vi "LSMcontroller_v57.vi"() -> ()   [LabVIEW 2015] (continued)
      # "Look in disabled \nchannelselect example next to this\nto understand how channels get propagated \nthrough the progam\n\nthe configuration file contains all\navailable channels in an array.\nat the start of the program lists of available \ninput channels and  menu rings of available output channels are loaded from here.\n\nif you add channels to record from/output to, make sure to expand the channel array in config.\n\nOnce the lists and rings are loaded, items in the list can be selected via click and  shift-click.\nThe ao channels in the ring are added one by one, with a defined waveform.\n\nPropagating through the program in the 2p param buffers are only 4 arrays of numbers, which are the indices of the selected channels from the list in order. \nThus, the index in the active channels array DOES NOT tell you which channel it represents: the actual CONTENT/NUMBER at a particular index in the active channels arrays tells you which channel it represents, since that number is the index in the fixed channel array in config."
      n2 = stacked-sequence {
        frame #0 {
          n3 = call "lifetimeparameters.vi"("command"="clear") -> ()  [unwired: 1 in, 1 out]
          n4 = call "2pparameters.vi"("command"="clear") -> ()  [unwired: 1 in, 1 out]
        }
        frame #1 {
          w39 = TRUE ("auto shutter")
          n5 = call "2pparameters.vi"("command"="get") -> ("params out"=w41:T12)  [unwired: 1 in]
          n6 = Bundle By Name(cluster=w41, "autoshutter"=w39, "auto OD"=w39) -> (w40:T12)
          n7 = local write "auto shutter"(w39) -> ()
          n8 = local write "auto OD"(w39) -> ()
          n9 = call "2pparameters.vi"("Params in"=w40, "command"="set") -> ()  [unwired: 1 out]
        }
        frame #2 {
          # "Disabled Thorlabs Zstage;\nneeds to be replaced by PI code"
          # "Initialize Z-axis controller: Thorlabs MTS25-Z8"
          n10 = disable-structure shown="Disabled" {
            frame Disabled {
              n11 = call "Z-ControllerInterFace.vi"() -> ("motorref"=w45:refnum<k7>)  [unwired: 1 in]
              n12 = call "setmotorparam.vi"("Automation Refnum in"=w45) -> ("motorref out"=w46:refnum<k7>)
              n13 = call "2pparameters.vi"("command"="get") -> ("params out"=w49:T12)  [unwired: 1 in]
              n14 = Bundle By Name(cluster=w49, "motorref"=w46) -> (w50:T12)
              n15 = call "2pparameters.vi"("Params in"=w50, "command"="set") -> ()  [unwired: 1 out]
            }
            frame Enabled {
            }
          }
          n16 = local write "Thorlabs Zstage disabled"(TRUE ("64bit disabled")) -> ()
        }
        frame #3 {
          n17 = call "2pparameters.vi"("command"="get") -> ("params out"=w53:T12)  [unwired: 1 in]
          n18 = Bundle By Name(cluster=w53, "type"="X-Y-t movie") -> (w55:T12)
          n19 = call "2pparameters.vi"("Params in"=w55, "command"="set") -> ()  [unwired: 1 out]
        }
      }
      n20 = property on="Exit" class="Bool (strict)"("Val(Sgnl)"=w24) -> ()  [unwired: 2 in, 2 out]
      n21 = property on="Start" class="Bool (strict)"("Val(Sgnl)"=w24) -> ()  [unwired: 2 in, 2 out]
      n22 = property on="Stop" class="Bool (strict)"("Val(Sgnl)"=w24) -> ()  [unwired: 2 in, 2 out]
      n23 = property on="Start" class="Bool (strict)"("Visible"=TRUE, "DisabledEnum"=T8."Enabled" ("Disabled")) -> ()  [unwired: 2 in, 2 out]
      n24 = property on="ROI" class="Bool (strict)"("DisabledEnum"=T8."Enabled" ("Disabled")) -> ()  [unwired: 2 in, 2 out]
      n25 = property on="ROI" class="Bool (strict)"("Value"=FALSE ("ROI")) -> ()  [unwired: 2 in, 2 out]
      n26 = property on="ROI" class="Bool (strict)"("Visible"=TRUE) -> ()  [unwired: 2 in, 2 out]
      n27 = local read "Measurement"() -> (w12:T5)
      n28 = flat-sequence {
        frame #0 {
          n29 = call "configuration.vi"("command"="set") -> ()  [unwired: 2 in, 2 out]
        }
        frame #1 {
          w57 = u16 1 items=["OD 0"=1, "OD 0.5"=2, "OD 1"=3, "OD 2"=4, "OD 3"=5, "OD 4"=6] ("New ODfilt")
          n30 = call "configuration.vi"("command"="get") -> ("config out"=w60:T13)  [unwired: 2 in, 1 out]
          n31 = local read "ODfilt"() -> (w58:u16)
          n32 = Unbundle By Name(w60) -> ("master data dir"=→"data dir":path)
          n33 = call "filterwheelcontrol_nothorlabslib.vi"("Current OD filt"=w57, "New ODfilt"=w58) -> ()  [unwired: 1 in]
        }
        frame #2 {
          n34 = call "configuration.vi"("command"="get") -> ("config out"=w64:T13)  [unwired: 2 in, 1 out]
          n35 = Unbundle By Name(w64) -> ("AI names"=w63:string[], "CI names"=w62:string[])
          n36 = property on="AI channels" class="LstBox (strict)"("Item Names"=w63) -> ()  [unwired: 2 in, 2 out]
          n37 = property on="CI channels" class="LstBox (strict)"("Item Names"=w62) -> ()  [unwired: 2 in, 2 out]
        }
        frame #3 {
          n38 = call "configuration.vi"("command"="get") -> ("config out"=w73:T13)  [unwired: 2 in, 1 out]
          n39 = Unbundle By Name(w73) -> ("AO names"=w69:string[], "DO names"=w68:string[])
          n40 = call "fill channelselector from array.vi"("channel  names"=w69) -> ("channel selector string and values"=w71:cluster{"String":string, "Value":u16}[])
          n41 = Build Array (concatenate)(w69, w68) -> (w67:string[])
          n42 = call "fill channelselector from array.vi"("channel  names"=w68) -> ("channel selector string and values"=w70:cluster{"String":string, "Value":u16}[])
          n43 = property on="AO channels" class="Ring (strict)"("StringsAndValues[]"=w71) -> ()  [unwired: 2 in, 2 out]
          n44 = call "fill channelselector from array.vi"("channel  names"=w67) -> ("channel selector string and values"=w66:cluster{"String":string, "Value":u16}[])
          n45 = property on="DO channels" class="Ring (strict)"("StringsAndValues[]"=w70) -> ()  [unwired: 2 in, 2 out]
          n46 = property on="refwf" class="Ring (strict)"("StringsAndValues[]"=w66) -> ()  [unwired: 2 in, 2 out]
        }
      }
      n47 = case shown="\"Lifetime (point)\", \"Lifetime (scan)\"" w12 {
        frame "Lifetime (point)", "Lifetime (scan)" {
          n48 = property on="Init" class="Bool (strict)"("Visible"=TRUE, "DisabledEnum"=T8."Enabled" ("Disabled")) -> ()  [unwired: 2 in, 2 out]
          n49 = property on="Start" class="Bool (strict)"("Visible"=FALSE, "DisabledEnum"=T8."Disabled and Grayed Out" ("Disabled")) -> ()  [unwired: 2 in, 2 out]
        }
        frame "X-Y-t movie", Default {
        }
      }
      n50 = call "seterrors.vi"("error IO"=errorcluster {"status"=FALSE, "code"=0, "source"=""}) -> ()
      n51 = property on="Stop" class="Bool (strict)"("Visible"=FALSE, "DisabledEnum"=T8."Disabled and Grayed Out" ("Disabled")) -> ()  [unwired: 2 in, 2 out]
      n52 = property on="Init" class="Bool (strict)"("Visible"=FALSE, "DisabledEnum"=T8."Disabled and Grayed Out" ("Disabled")) -> ()  [unwired: 2 in, 2 out]
      n53 = Current VI's Path() -> (path=w10:path)
      n54 = Strip Path(path=w10) -> (stripped path=w11:path)  [unwired: 1 out]
      n55 = Build Path(base path=w11, name or relative path="LaserControl.vi") -> (appended path=w9:path)
      n56 = call "loadcolormaps.vi"() -> ()  [unwired: 12 in]
      n57 = stacked-sequence {
        frame #0 {
          n58 = call "waveformsDObuffer.vi"("command"="clear") -> ()  [unwired: 1 in, 1 out]
          n59 = call "waveformsAObuffer.vi"("command"="clear") -> ()  [unwired: 1 in, 1 out]
        }
        frame #1 {
          n60 = call "Used AO lines.vi"() -> ("used AO names"=w27:string[], "used AO lines"=w29:tag[])  [unwired: 2 in]
          n61 = control-ref of="Analog Lines Plot"() -> (w28:refnum<vi>)
          n62 = local write "Analog Used Lines"(w29) -> ()
          n63 = local write "Analog Used Names"(w27) -> ()
          n64 = call "prepAOWaveplot.vi"("WaveformGraph in"=w28, "Analog Used Names"=w27) -> ()  [unwired: 1 in]
          n65 = control-ref of="Digital Lines Plot"() -> (w30:refnum<vi>)
          n66 = call "Used DO lines.vi"() -> ("used DO names"=w31:string[], "used DO lines"=w32:tag[])  [unwired: 2 in]
          n67 = local write "Digital Used Lines"(w32) -> ()
          n68 = local write "Digital Used Names"(w31) -> ()
          n69 = call "prepDOWaveplot.vi"("DigitalGraph in"=w30, "used DO names"=w31) -> ()  [unwired: 1 in]
        }
      }
      n70 = Open VI Reference(type specifier VI Refnum (for type only)=refnum<vi> refnum, vi path=w9, options=128) -> (vi reference=w2:refnum<vi>, error out=w6:errorcluster)  [unwired: 3 in]
      n71 = call-by-ref "Start Asynchronous Call"(reference=w2, error in=w6) -> (reference out=w7:refnum<vi>, error out=w5:errorcluster)  [unwired: 12 in]
      n72 = Close Reference(reference=w7, error in (no error)=w5) -> ()  [unwired: 1 out]
      n73 = disable-structure shown="Enabled" {
        frame Disabled {
          n74 = call "channelselectexample.vi"() -> ()  [unwired: 12 in]
        }
        frame Enabled {
        }
      }
      "ROI Type" <- w15
    }
    frame #2 {
      n75 = while {
        stop <- w2050 stop-if-true
        n76 = event shown="[15] \"readpatch\": Value Change" {
          selector: _ -> [_ _ _ _ _ _ _ _ _ _ _ _ _ _ _ _ _ _ _ _ _ _ _ _ _ _ _ _ _ _ _ _ _ _ _ _ _ _ _ _ _]
          dyn-events: _ -> [_ _ _ _ _ _ _ _ _ _ _ _ _ _ _ _ _ _ _ _ _ _ _ _ _ _ _ _ _ _ _ _ _ _ _ _ _ _ _ _ _]
          timeout: _ -> [_ _ _ _ _ _ _ _ _ _ _ _ _ _ _ _ _ _ _ _ _ _ _ _ _ _ _ _ _ _ _ _ _ _ _ _ _ _ _ _ _]
          tunnel: [_ _ _ _ _ _ _ _ _ _ _ _ _ _ _ _ _ _ _ _ _ _ _ _ _ _ _ _ _ _ _ _ _ _ _ _ _ _ _ _ "Exit"] -> w2050
          event "Start": Value Change {
            n77 = event-data() -> ()  [unwired: 1 in, 5 out]
            n78 = local read "Start"() -> (w2051:bool)
            n79 = case shown="True" w2051 {
              frame False {
              }
              frame True {
                # "X"
                # "Y"
                n80 = local read "Measurement"() -> (w2052:T5)
                n81 = case shown="\"Timetrace\", \"Lifetime (contour)\"" w2052 {
                  frame "X-Y-t movie", "X-Y-Z stack", "Lifetime (scan)" {
                    n82 = stacked-sequence {
                      seq-local: [_ w2094 _ _ _ _ _ _ _ _ _ _ _] -> [_ _ _ w2947 _ _ _ w2979 w3156 _ _ w3566 _]
                      seq-local: [_ w2092 _ _ _ _ _ _ _ _ _ _ _] -> [_ _ _ _ _ _ _ _ _ _ w3256 _ _]
                      seq-local: [_ w2091 _ _ _ _ _ _ _ _ _ _ _] -> [_ _ _ _ _ _ _ _ _ _ w3255 _ _]
                      seq-local: [_ w2090 _ _ _ _ _ _ _ _ _ _ _] -> [_ _ _ _ _ _ _ _ _ _ w3254 _ _]
                      seq-local: [_ w2089 _ _ _ _ _ _ _ _ _ _ _] -> [_ _ _ _ _ _ _ _ _ _ w3253 _ _]
                      seq-local: [_ w2088 _ _ _ _ _ _ _ _ _ _ _] -> [_ _ _ _ _ _ _ _ _ _ w3252 _ _]
                      seq-local: [_ w2087 _ _ _ _ _ _ _ _ _ _ _] -> [_ _ _ _ _ _ _ _ _ _ w3251 _ _]
                      seq-local: [_ w2086 _ _ _ _ _ _ _ _ _ _ _] -> [_ _ _ _ _ _ _ _ _ _ w3246 _ _]
                      seq-local: [_ w2085 _ _ _ _ _ _ _ _ _ _ _] -> [_ _ _ _ _ _ _ _ _ _ w3245 _ _]
                      seq-local: [_ w2084 _ _ _ _ _ _ _ _ _ _ _] -> [_ _ _ _ _ _ _ _ _ _ w3250 _ _]
                      seq-local: [_ w2083 _ _ _ _ _ _ _ _ _ _ _] -> [_ _ _ _ _ _ _ _ _ _ w3249 _ _]
                      seq-local: [_ w2081 _ _ _ _ _ _ _ _ _ _ _] -> [_ _ _ _ _ _ _ _ _ _ w3244 _ _]
                      seq-local: [_ w2082 _ _ _ _ _ _ _ _ _ _ _] -> [_ _ _ _ _ _ _ _ _ _ w3243 _ _]
                      seq-local: [_ w2080 _ _ _ _ _ _ _ _ _ _ _] -> [_ _ _ _ _ _ _ _ _ _ w3247 _ _]
                      seq-local: [_ w2079 _ _ _ _ _ _ _ _ _ _ _] -> [_ _ _ _ _ _ _ _ _ _ w3248 _ _]
                      frame #0 {
                        w2053 = u16 0 items=["Image", "Rectangle", "Circle", "Freeform Boundary", "Freeform Interior", "Ellipse Boundary", "Line"] ("ROI Type")
                        n83 = local read "finite samples"() -> (w2054:bool)
                        n84 = case shown="True" w2054 {
                          frame False {
                          }
                          frame True {
                            n85 = local read "# of frames"() -> (w2055:i32)
                            n86 = Greater?(x=w2055, y=999) -> (0:w2056:bool)
                            n87 = case shown="True" w2056 {
                              tunnel: w2055 -> [_ w2060]
                              frame False {
                              }
                              frame True {
                                n88 = flat-sequence {
                                tunnel: w2060 -> [w2061]
                                tunnel: [w2062] -> w2059
                                tunnel: [w2061] -> w2058
                                tunnel: w2059 -> [w2074]
                                tunnel: w2058 -> [w2073]
                                frame #0 {
                                n89 = Number To Decimal String(number=w2061) -> (decimal integer string=w2066:string)  [unwired: 1 in]
                                n90 = Concatenate Strings("Yes: record " ("Left Button Text (\"Yes\")"), w2066, " frames" ("string")) -> (w2067:string)
                                n91 = Concatenate Strings("# of frames is " ("message"), w2066, ". Did you mean to do that?" ("string")) -> (w2069:string)
                                n92 = call <vilib>:"Three Button Dialog.vi"("Allow user to close window? (TRUE)"=FALSE, "Right Button Text (\"Cancel\")"="no: record 10 frames" ("Right Button Text (\"Cancel\")"), "Center Button Text (\"No\")"="No: record 1 frame" ("Center Button Text (\"No\")"), "Left Button Text (\"Yes\")"=w2067, "message"=w2069) -> ("Which Button?"=w2062:T14)  [unwired: 6 in]
                                }
                                frame #1 {
                                n93 = case shown="\"Window Close\"" w2074 {
                                tunnel: w2073 -> [w2075 _ _ _]
                                frame "Left Button" {
                                n94 = local write "# of frames"(w2075) -> ()
                                }
                                frame "Center Button", Default {
                                n95 = local write "# of frames"(1 ("# of frames")) -> ()
                                }
                                frame "Right Button" {
                                n96 = local write "# of frames"(10 ("# of frames")) -> ()
                                }
                                frame "Window Close" {
                                n97 = local write "# of frames"(1 ("# of frames")) -> ()
                                }
                                }
                                }
                                }
                              }
                            }
                          }
                        }
                        n98 = local write "ROI Type"(w2053) -> ()
                      }
                      frame #1 {
                        # "change active waveform numbers array"
                        n99 = local read "save\ndata"() -> (w2093:bool)
                        n100 = Get Date/Time In Seconds() -> (seconds since 1Jan1904=w2095:timestamp)
                        n101 = case shown="True" w2093 {
                          tunnel: w2095 -> [w2096 w2098]
                          tunnel: [w2096 w2097] -> w2094
                          frame False {
                          }
                          frame True {
                            n102 = call "createdatafolder.vi"("timestamp in"=w2098) -> ("current data path"=w2099:path, "timestamp out"=w2097:timestamp)
                            n103 = local write "data dir"(w2099) -> ()
                          }
                        }
                        n104 = stacked-sequence {
                          tunnel: w2094 -> [_ w2106 _ _ _ _ _ _ _ _]
                          tunnel: [_ _ _ _ _ w2249 _ _ _ _] -> w2092
                          tunnel: [_ _ _ _ _ w2248 _ _ _ _] -> w2091
                          tunnel: [_ _ _ _ _ w2247 _ _ _ _] -> w2090
                          tunnel: [_ _ _ _ _ w2246 _ _ _ _] -> w2089
                          tunnel: [_ _ _ _ _ w2245 _ _ _ _] -> w2088
                          tunnel: [_ _ _ _ _ w2244 _ _ _ _] -> w2087
                          tunnel: [_ _ _ _ _ w2243 _ _ _ _] -> w2086
                          tunnel: [_ _ _ _ _ w2242 _ _ _ _] -> w2085
                          tunnel: [_ _ _ _ _ w2241 _ _ _ _] -> w2084
                          tunnel: [_ _ _ _ _ w2240 _ _ _ _] -> w2083
                          tunnel: [_ _ _ _ _ w2239 _ _ _ _] -> w2082
                          tunnel: [_ _ _ _ _ w2238 _ _ _ _] -> w2081
                          tunnel: [_ _ _ _ _ w2237 _ _ _ _] -> w2080
                          tunnel: [_ _ _ _ _ w2236 _ _ _ _] -> w2079
                          frame #0 {
                            n105 = local read "AI channels"() -> (w2105:i32[])
                            n106 = local read "CI channels"() -> (w2104:i32[])
                            n107 = call "2pparameters.vi"("command"="get") -> ("params out"=w2102:T12)  [unwired: 1 in]
                            n108 = Bundle By Name(cluster=w2102, "aAI"=w2105, "aCI"=w2104) -> (w2103:T12)
                            n109 = call "2pparameters.vi"("Params in"=w2103, "command"="set") -> ()  [unwired: 1 out]
                          }
                          frame #1 {
                            n110 = local read "Vy-min ref"() -> (w2110:dbl)
                            n111 = local read "Vy-max ref"() -> (w2111:dbl)
                            n112 = local read "Angle ref"() -> (w2109:dbl)
                            n113 = local read "Vx-min ref"() -> (w2112:dbl)
                            n114 = local write "counts"(0 ("counts")) -> ()
                            n115 = local write "graphtab"(T6."image" ("graphtab")) -> ()
                            n116 = local read "Vx-max ref"() -> (w2113:dbl)
                            n117 = property on="Stop" class="Bool (strict)"("Visible"=TRUE, "DisabledEnum"=T8."Enabled" ("Disabled")) -> ()  [unwired: 2 in, 2 out]
                            n118 = property on="Start" class="Bool (strict)"("Visible"=FALSE, "DisabledEnum"=T8."Disabled and Grayed Out" ("Disabled")) -> ()  [unwired: 2 in, 2 out]
                            n119 = script code="Xic=(ximax+ximin)./2;\nYic=(yimax+yimin)./2;\nximin=ximin-Xic;\nymin=ymin-Yic;\nxirmin=ximin.*cos(pi/180.*phi)+yimin.*sin(pi./180.*phi)+Xic;\nyirmin=-ximin.*sin(pi./180.*phi)+yimin.*cos(pi./180.*phi)+Yic;"("ximax"=w2113, "ximin"=w2112, "yimax"=w2111, "yimin"=w2110, "phi"=w2109) -> ("xirmin"=w2108:dbl, "yirmin"=w2107:dbl)  [unwired: 1 in, 1 out]
                            n120 = stacked-sequence {
                              tunnel: w2106 -> [_ w2138 _]
                              frame #0 {
                                n121 = local read "Measurement"() -> (w2120:T5)
                                n122 = case shown="\"X-Y-Z stack\"" w2120 {
                                frame "X-Y-t movie", Default {
                                n123 = call "2pparameters.vi"("command"="get") -> ("params out"=w2123:T12)  [unwired: 1 in]
                                n124 = Bundle By Name(cluster=w2123, "type"="X-Y-t movie") -> (w2121:T12)
                                n125 = call "2pparameters.vi"("Params in"=w2121, "command"="set") -> ()  [unwired: 1 out]
                                }
                                frame "X-Y-Z stack" {
                                n126 = call "2pparameters.vi"("command"="get") -> ("params out"=w2128:T12)  [unwired: 1 in]
                                n127 = Bundle By Name(cluster=w2128, "type"="X-Y-Z stack") -> (w2126:T12)
                                n128 = call "2pparameters.vi"("Params in"=w2126, "command"="set") -> ()  [unwired: 1 out]
                                }
                                frame "Lifetime (scan)" {
                                n129 = call "2pparameters.vi"("command"="get") -> ("params out"=w2133:T12)  [unwired: 1 in]
                                n130 = Bundle By Name(cluster=w2133, "type"="Lifetime (scan)") -> (w2131:T12)
                                n131 = call "2pparameters.vi"("Params in"=w2131, "command"="set") -> ()  [unwired: 1 out]
                                }
                                }
                              }
                              frame #1 {
                                n132 = Format Date/Time String(time format string (%c)="%Y%m%d", seconds (now)=w2138) -> (date/time string=w2137:string)  [unwired: 1 in]
                                n133 = Format Date/Time String(time format string (%c)="%H%M%S", seconds (now)=w2138) -> (date/time string=w2136:string)  [unwired: 1 in]
                                n134 = call "2pparameters.vi"("command"="get") -> ("params out"=w2142:T12)  [unwired: 1 in]
                                n135 = Bundle By Name(cluster=w2142, "date"=w2137, "time"=w2136) -> (w2141:T12)
                                n136 = call "2pparameters.vi"("Params in"=w2141, "command"="set") -> ()  [unwired: 1 out]
                              }
                              frame #2 {
                                n137 = call "configuration.vi"("command"="get") -> ("config out"=w2152:T13)  [unwired: 2 in, 1 out]
                                n138 = Unbundle By Name(w2152) -> ("CI names"=w2153:string[], "AI names"=w2154:string[])
                                n139 = call "2pparameters.vi"("command"="get") -> ("params out"=w2148:T12)  [unwired: 1 in]
                                n140 = Unbundle By Name(w2148) -> ("aCI"=w2149:i32[], "aAI"=w2150:i32[])
                                n141 = for {
                                tunnel: w2149 -> [w2164] mode=indexing
                                tunnel: w2153 -> [w2165]
                                tunnel: [w2163] -> w2155 mode=indexing
                                n142 = Index Array(array=w2165, index=w2164) -> (element=w2163:string)
                                }
                                n143 = for {
                                tunnel: w2150 -> [w2161] mode=indexing
                                tunnel: w2154 -> [w2162]
                                tunnel: [w2160] -> w2156 mode=indexing
                                n144 = Index Array(array=w2162, index=w2161) -> (element=w2160:string)
                                }
                                n145 = Build Array (concatenate)(w2155, w2156) -> (w2146:string[])
                                n146 = for {
                                tunnel: w2146 -> [w2158] mode=indexing
                                tunnel: [w2157] -> w2145 mode=indexing
                                i -> [w2159]
                                n147 = Bundle("String"=w2158, w2159) -> (w2157:cluster{"String":string, i32})  [unwired: 1 in]
                                }
                                n148 = property on="image1list" class="Ring (strict)"("StringsAndValues[]"=w2145) -> ()  [unwired: 2 in, 2 out]
                                n149 = property on="image2list" class="Ring (strict)"("StringsAndValues[]"=w2145) -> ()  [unwired: 2 in, 2 out]
                              }
                            }
                            n150 = call "setposition.vi"("Vy"=w2107, "Vx"=w2108) -> ()  [unwired: 1 in]
                          }
                          frame #2 {
                            n151 = call "X-array-databuffer.vi"("command"=enum16{"get", "set", "clear", "append"}."clear") -> ()  [unwired: 3 in, 2 out]
                            n152 = call "Y-array-databuffer.vi"("command"=enum16{"get", "set", "clear", "append"}."clear") -> ()  [unwired: 3 in, 2 out]
                            n153 = call "2pparameters.vi"("command"="get") -> ("params out"=w2168:T12)  [unwired: 1 in]
                            n154 = Unbundle By Name(w2168) -> ("autoshutter"=w2169:bool, "auto OD"=w2166:bool)
                            n155 = call "allAI-temp_img.vi"("command"=enum16{"get", "set", "clear", "append"}."clear") -> ()  [unwired: 3 in, 2 out]
                            n156 = case shown="True" w2166 {
                              frame False {
                              }
                              frame True {
                                n157 = call "configuration.vi"("command"="get") -> ("config out"=w2177:T13)  [unwired: 2 in, 1 out]
                                n158 = Unbundle By Name(w2177) -> ("image OD"=w2178:u16)
                                n159 = local read "ODfilt"() -> (w2175:u16)
                                n160 = call "filterwheelcontrol_nothorlabslib.vi"("Current OD filt"=w2175, "New ODfilt"=w2178) -> ()  [unwired: 1 in]
                              }
                            }
                            n161 = case shown="True" w2169 {
                              frame False {
                              }
                              frame True {
                                n162 = call "shuttercontrol.vi"("command"="close") -> ()  [unwired: 1 in, 1 out]
                              }
                            }
                            n163 = call "CH1-temp.vi"("command"=enum16{"get", "set", "clear", "add row"}."clear") -> ()  [unwired: 3 in, 2 out]
                            n164 = call "CH2-temp.vi"("command"=enum16{"get", "set", "clear", "add row"}."clear") -> ()  [unwired: 3 in, 2 out]
                          }
                          frame #3 {
                            n165 = local read "avpp"() -> (w2212:i32)
                            n166 = local read "Angle ref"() -> (w2211:dbl)
                            n167 = local read "ROI Type"() -> (w2210:u16)
                            n168 = local read "xpixels ref"() -> (w2207:i32)
                            n169 = local read "Vx-min ref"() -> (w2206:dbl)
                            n170 = local read "Vx-max ref"() -> (w2205:dbl)
                            n171 = local read "ypixels ref"() -> (w2203:i32)
                            n172 = local read "Vy-min ref"() -> (w2204:dbl)
                            n173 = local read "Vy-max ref"() -> (w2200:dbl)
                            n174 = local read "Sampling rate"() -> (w2194:dbl)
                            n175 = local read "finite samples"() -> (w2195:bool)
                            n176 = local read "continuous"() -> (w2198:bool)
                            n177 = local read "wavdet"() -> (w2199:bool)
                            n178 = local read "# of frames"() -> (w2197:i32)
                            n179 = local read "maxbufferAI"() -> (w2196:i32)
                            n180 = local read "Override AI buffer"() -> (w2180:bool)
                            n181 = call "2pparameters.vi"("command"="get") -> ("params out"=w2209:T12)  [unwired: 1 in]
                            n182 = Bundle By Name(cluster=w2209, "avpp"=w2212, "Angle Img"=w2211, "Xpixels Img"=w2207, "Vx-min Img"=w2206, "VX-max Img"=w2205, "Ypixels Img"=w2203, "Vy-min Img"=w2204, "Vy-max Img"=w2200, "srate"=w2194, "srate Img"=w2194, "finite"=w2195, "cont"=w2198, "wavdet"=w2199, "measpoints"=w2197, "maxbufferAI"=w2196, "Drawing Mode"=w2210, "Vz-reset"=0.0, "AIoverride"=w2180) -> (w2201:T12)
                            n183 = call "2pparameters.vi"("Params in"=w2201, "command"="set") -> ()  [unwired: 1 out]
                            n184 = local read "Vholding (mV)"() -> (w2183:sgl)
                            n185 = local read "Current Clamp"() -> (w2189:bool)
                            n186 = local read "Voltage Clamp"() -> (w2188:bool)
                            n187 = local read "OCgain"() -> (w2184:sgl)
                            n188 = local read "CC_ICgain"() -> (w2187:dbl)
                            n189 = local read "holdon"() -> (w2182:bool)
                            n190 = call "patchparameters.vi"("command"="get") -> ("Params out"=w2191:T15)  [unwired: 1 in]
                            n191 = Bundle By Name(cluster=w2191, "VC"=w2188, "CC"=w2189, "CC_icg (pA/mv)"=w2187, "VC_icg (mV/mV)"=sgl 10.0, "OCG (mV/pA)"=w2184, "OVG (mV/mV)"=0.1, "Vhold (mV)"=w2183, "holdon"=w2182) -> (w2190:T15)
                            n192 = call "patchparameters.vi"("Params in"=w2190, "command"="set") -> ()  [unwired: 1 out]
                          }
                          frame #4 {
                            # "Generate Waveforms for Scanning Mirrors"
                            n193 = call "2pparameters.vi"("command"="get") -> ("params out"=w2227:T12)  [unwired: 1 in]
                            n194 = Unbundle By Name(w2227) -> ("srate Img"=w2226:sgl, "Angle Img"=w2225:dbl, "VX-max Img"=w2224:dbl, "Vx-min Img"=w2223:dbl, "Xpixels Img"=w2222:i32, "Ypixels Img"=w2221:i32, "Vy-max Img"=w2220:dbl, "Vy-min Img"=w2219:dbl, "Drawing Mode"=w2218:u16)
                            n195 = call "ROI-databuffer.vi"("command"=enum16{"get", "set", "clear", "append"}."get") -> ("array out"=w2217:cluster{"x":sgl, "y":sgl}[])  [unwired: 4 in]
                            n196 = call "ScanningWaveform_v4.vi"("Vy-min"=w2219, "Vy-max"=w2220, "yPixels/tPixels"=w2221, "xPixels/rPixels"=w2222, "Vx-min"=w2223, "Vx-max"=w2224, "Drawing Mode"=w2218, "Angle"=w2225, "AOrate"=w2226, "Points"=w2217) -> ("numPixels"=w2213:dbl, "Y-WaveArray"=w2216:dbl[], "P"=w2214:dbl, "X-WaveArray"=w2215:dbl[])  [unwired: 6 in]
                            n197 = call "2pparameters.vi"("command"="get") -> ("params out"=w2235:T12)  [unwired: 1 in]
                            n198 = call "Y-array-databuffer.vi"("array in"=w2216, "command"=enum16{"get", "set", "clear", "append"}."set") -> ()  [unwired: 2 in, 2 out]
                            n199 = call "X-array-databuffer.vi"("array in"=w2215, "command"=enum16{"get", "set", "clear", "append"}."set") -> ()  [unwired: 2 in, 2 out]
                            n200 = Bundle By Name(cluster=w2235, "P"=w2214, "sAOxy"=w2213) -> (w2232:T12)
                            n201 = call "2pparameters.vi"("Params in"=w2232, "command"="set") -> ()  [unwired: 1 out]
                          }
                          frame #5 {
                            # "rem2Ps"
                            # "A2Ps"
                            # "Al"
                            # "Rl"
                            n202 = stacked-sequence {
                              seq-local: [w2254 _ _ _ _ _ _ _ _ _ _] -> [_ w2366 _ w2421 _ w2501 _ _ _ _ _]
                              seq-local: [w2255 _ _ _ _ _ _ _ _ _ _] -> [_ w2367 w2377 _ w2470 _ _ _ _ _ _]
                              seq-local: [_ _ w2376 _ _ _ _ _ _ _ _] -> [_ _ _ _ w2464 _ _ _ _ _ _]
                              seq-local: [_ _ _ w2420 _ _ _ _ _ _ _] -> [_ _ _ _ _ w2500 _ _ _ _ _]
                              seq-local: [w2251 _ _ _ _ _ _ _ _ _ _] -> [_ w2363 _ _ _ _ _ _ w2686 w2754 _]
                              seq-local: [w2250 _ _ _ _ _ _ _ _ _ _] -> [_ w2362 _ _ _ _ _ _ w2687 w2755 _]
                              seq-local: [w2257 _ _ _ _ _ _ _ _ _ _] -> [_ _ _ _ _ _ w2539 _ w2685 w2753 _]
                              seq-local: [w2253 _ _ _ _ _ _ _ _ _ _] -> [_ w2361 _ _ _ _ w2538 w2606 _ _ _]
                              seq-local: [w2252 _ _ _ _ _ _ _ _ _ _] -> [_ w2360 _ _ _ _ w2537 w2605 _ _ _]
                              seq-local: [w2256 _ _ _ _ _ _ _ _ _ _] -> [_ _ _ _ _ _ w2536 w2604 _ _ _]
                              tunnel: [_ _ w2375 _ _ _ _ _ _ _ _] -> w2248
                              tunnel: [_ _ w2374 _ _ _ _ _ _ _ _] -> w2247
                              tunnel: [w2255 _ _ _ _ _ _ _ _ _ _] -> w2249
                              tunnel: [w2254 _ _ _ _ _ _ _ _ _ _] -> w2246
                              tunnel: [_ _ _ w2419 _ _ _ _ _ _ _] -> w2245
                              tunnel: [_ _ _ w2418 _ _ _ _ _ _ _] -> w2244
                              tunnel: [w2253 _ _ _ _ _ _ _ _ _ _] -> w2243
                              tunnel: [w2252 _ _ _ _ _ _ _ _ _ _] -> w2242
                              tunnel: [_ _ _ _ _ _ w2535 _ _ _ _] -> w2241
                              tunnel: [_ _ _ _ _ _ _ w2603 _ _ _] -> w2240
                              tunnel: [w2251 _ _ _ _ _ _ _ _ _ _] -> w2239
                              tunnel: [w2250 _ _ _ _ _ _ _ _ _ _] -> w2238
                              tunnel: [_ _ _ _ _ _ _ _ w2684 _ _] -> w2237
                              tunnel: [_ _ _ _ _ _ _ _ _ w2752 _] -> w2236
                              frame #0 {
                                # "for a next version, give ome thought to\nthe possibilit of intermittently updating the\nwaveforms. it will have to be a calculation\nbased on speed of CPU and program on the one hand\nand length of measurement on the other. but then it should be possible, in principle, to \nupdate the waveform on the fly and that way cut up a longer measurement in smaller parts."
                                # "Y"
                                # "X"
                                n203 = stacked-sequence {
                                tunnel: [w2258 _ _ _] -> w2255
                                tunnel: [_ w2270 _ _] -> w2254
                                tunnel: [_ _ _ w2327] -> w2250
                                tunnel: [_ _ _ w2326] -> w2251
                                tunnel: [_ _ _ w2325] -> w2257
                                tunnel: [_ _ w2285 _] -> w2253
                                tunnel: [_ _ w2284 _] -> w2252
                                tunnel: [_ _ w2283 _] -> w2256
                                frame #0 {
                                n204 = call "configuration.vi"("command"="get") -> ("config out"=w2260:T13)  [unwired: 2 in, 1 out]
                                n205 = Unbundle By Name(w2260) -> ("Voltage to Xgalvo"=w2259:i32)
                                n206 = call "2pparameters.vi"("command"="get") -> ("params out"=w2264:T12)  [unwired: 1 in]
                                n207 = in-place {
                                in-place-border: w2259 -> [w2269]
                                in-place-border: [w2266] -> w2258
                                n208 = in-place-cluster #1(w2264) -> ("aAO"=w2268:u32[])
                                n209 = call "add channel to active arrayv2.vi"("line array in"=w2268, "line to add"=w2269) -> ("line array out"=w2267:u32[], "addition"=w2266:bool)  [unwired: 1 out]
                                n210 = in-place-cluster #1("aAO"=w2267) -> (w2262:T12)
                                }
                                n211 = call "2pparameters.vi"("Params in"=w2262, "command"="set") -> ()  [unwired: 1 out]
                                }
                                frame #1 {
                                n212 = call "configuration.vi"("command"="get") -> ("config out"=w2272:T13)  [unwired: 2 in, 1 out]
                                n213 = Unbundle By Name(w2272) -> ("Voltage to Ygalvo"=w2271:i32)
                                n214 = call "2pparameters.vi"("command"="get") -> ("params out"=w2276:T12)  [unwired: 1 in]
                                n215 = in-place {
                                in-place-border: w2271 -> [w2281]
                                in-place-border: [w2278] -> w2270
                                n216 = in-place-cluster #2(w2276) -> ("aAO"=w2280:u32[])
                                n217 = call "add channel to active arrayv2.vi"("line array in"=w2280, "line to add"=w2281) -> ("line array out"=w2279:u32[], "addition"=w2278:bool)  [unwired: 1 out]
                                n218 = in-place-cluster #2("aAO"=w2279) -> (w2274:T12)
                                }
                                n219 = call "2pparameters.vi"("Params in"=w2274, "command"="set") -> ()  [unwired: 1 out]
                                }
                                frame #2 {
                                n220 = call "2pparameters.vi"("command"="get") -> ("params out"=w2287:T12)  [unwired: 1 in]
                                n221 = Unbundle By Name(w2287) -> ("autoshutter"=w2286:bool, "wavdet"=w2282:bool)
                                n222 = case shown="True" w2286 {
                                tunnel: [w2292 w2312] -> w2285
                                tunnel: [w2291 FALSE ("removal")] -> w2284
                                tunnel: [w2290 w2310] -> w2283
                                tunnel: w2282 -> [w2289 _]
                                frame False {
                                n223 = case shown="False" w2289 {
                                tunnel: [FALSE ("addition") FALSE ("addition")] -> w2292
                                tunnel: [w2294 FALSE ("removal")] -> w2291
                                tunnel: [w2293 _] -> w2290
                                frame False {
                                n224 = call "configuration.vi"("command"="get") -> ("config out"=w2300:T13)  [unwired: 2 in, 1 out]
                                n225 = Unbundle By Name(w2300) -> ("2P shutter"=w2297:i32)
                                n226 = call "2pparameters.vi"("command"="get") -> ("params out"=w2298:T12)  [unwired: 1 in]
                                n227 = in-place {
                                in-place-border: w2297 -> [w2307]
                                in-place-border: [w2304] -> w2294
                                in-place-border: [w2303] -> w2293
                                n228 = in-place-cluster #3(w2298) -> ("aDO"=w2306:u32[])
                                n229 = call "remove channel from active arrayv2.vi"("line array in"=w2306, "line to remove"=w2307) -> ("line array out"=w2305:u32[], "removal"=w2304:bool, "index"=w2303:i32)
                                n230 = in-place-cluster #3("aDO"=w2305) -> (w2295:T12)
                                }
                                n231 = call "2pparameters.vi"("Params in"=w2295, "command"="set") -> ()  [unwired: 1 out]
                                }
                                frame True {
                                }
                                }
                                }
                                frame True {
                                n232 = call "configuration.vi"("command"="get") -> ("config out"=w2314:T13)  [unwired: 2 in, 1 out]
                                n233 = call "2pparameters.vi"("command"="get") -> ("params out"=w2318:T12)  [unwired: 1 in]
                                n234 = Unbundle By Name(w2314) -> ("2P shutter"=w2313:i32)
                                n235 = in-place {
                                in-place-border: w2313 -> [w2324]
                                in-place-border: [w2321] -> w2312
                                in-place-border: [w2320] -> w2310
                                n236 = in-place-cluster #4(w2318) -> ("aDO"=w2323:u32[])
                                n237 = call "add channel to active arrayv2.vi"("line array in"=w2323, "line to add"=w2324) -> ("line array out"=w2322:u32[], "addition"=w2321:bool, "index"=w2320:i32)
                                n238 = in-place-cluster #4("aDO"=w2322) -> (w2316:T12)
                                }
                                n239 = call "2pparameters.vi"("Params in"=w2316, "command"="set") -> ()  [unwired: 1 out]
                                }
                                }
                                }
                                frame #3 {
                                n240 = local read "Measurement"() -> (w2328:T5)
                                n241 = To Unsigned Long Integer(number=w2328) -> (unsigned 32bit integer=w2329:u32)
                                n242 = case shown="5..7" w2329 {
                                tunnel: [FALSE ("addition") w2347] -> w2327
                                tunnel: [w2332 FALSE ("removal")] -> w2326
                                tunnel: [w2330 w2345] -> w2325
                                frame 0..4, Default {
                                n243 = call "configuration.vi"("command"="get") -> ("config out"=w2338:T13)  [unwired: 2 in, 1 out]
                                n244 = Unbundle By Name(w2338) -> ("LT timestamp"=w2335:u32)
                                n245 = call "2pparameters.vi"("command"="get") -> ("params out"=w2336:T12)  [unwired: 1 in]
                                n246 = in-place {
                                in-place-border: w2335 -> [w2344]
                                in-place-border: [w2341] -> w2332
                                in-place-border: [w2340] -> w2330
                                n247 = in-place-cluster #5(w2336) -> ("aDO"=w2343:u32[])
                                n248 = call "remove channel from active arrayv2.vi"("line array in"=w2343, "line to remove"=w2344) -> ("line array out"=w2342:u32[], "removal"=w2341:bool, "index"=w2340:i32)
                                n249 = in-place-cluster #5("aDO"=w2342) -> (w2333:T12)
                                }
                                n250 = call "2pparameters.vi"("Params in"=w2333, "command"="set") -> ()  [unwired: 1 out]
                                }
                                frame 5..7 {
                                n251 = call "configuration.vi"("command"="get") -> ("config out"=w2353:T13)  [unwired: 2 in, 1 out]
                                n252 = Unbundle By Name(w2353) -> ("LT timestamp"=w2350:u32)
                                n253 = call "2pparameters.vi"("command"="get") -> ("params out"=w2351:T12)  [unwired: 1 in]
                                n254 = in-place {
                                in-place-border: w2350 -> [w2359]
                                in-place-border: [w2356] -> w2347
                                in-place-border: [w2355] -> w2345
                                n255 = in-place-cluster #6(w2351) -> ("aDO"=w2358:u32[])
                                n256 = call "add channel to active arrayv2.vi"("line array in"=w2358, "line to add"=w2359) -> ("line array out"=w2357:u32[], "addition"=w2356:bool, "index"=w2355:i32)
                                n257 = in-place-cluster #6("aDO"=w2357) -> (w2348:T12)
                                }
                                n258 = call "2pparameters.vi"("Params in"=w2348, "command"="set") -> ()  [unwired: 1 out]
                                }
                                }
                                }
                                }
                              }
                              frame #1 {
                                n259 = Or(x=w2366, y=w2367) -> (x .or. y?=w2365:bool)
                                n260 = case shown="True" w2365 {
                                frame False {
                                }
                                frame True {
                                # "update GUI"
                                n261 = call "Used AO lines.vi"() -> ("used AO names"=w2371:string[], "used AO lines"=w2373:tag[])  [unwired: 2 in]
                                n262 = control-ref of="Analog Lines Plot"() -> (w2372:refnum<vi>)
                                n263 = local write "Analog Used Lines"(w2373) -> ()
                                n264 = local write "Analog Used Names"(w2371) -> ()
                                n265 = call "prepAOWaveplot.vi"("WaveformGraph in"=w2372, "Analog Used Names"=w2371) -> ()  [unwired: 1 in]
                                }
                                }
                                n266 = Compound Arithmetic op=OR(w2363, w2362, w2361, w2360) -> (w2364:bool)
                                n267 = case shown="True" w2364 {
                                frame False {
                                }
                                frame True {
                                n268 = control-ref of="Digital Lines Plot"() -> (w2368:refnum<vi>)
                                n269 = call "Used DO lines.vi"() -> ("used DO names"=w2369:string[], "used DO lines"=w2370:tag[])  [unwired: 2 in]
                                n270 = local write "Digital Used Lines"(w2370) -> ()
                                n271 = local write "Digital Used Names"(w2369) -> ()
                                n272 = call "prepDOWaveplot.vi"("DigitalGraph in"=w2368, "used DO names"=w2369) -> ()  [unwired: 1 in]
                                }
                                }
                              }
                              frame #2 {
                                n273 = case shown="False" w2377 {
                                tunnel: [w2380 w2401] -> w2376
                                tunnel: [w2379 w2399] -> w2375
                                tunnel: [w2378 _] -> w2374
                                frame False {
                                n274 = stacked-sequence {
                                seq-local: [w2382 _] -> [_ w2395]
                                tunnel: [w2382 _] -> w2380
                                tunnel: [w2385 _] -> w2379
                                tunnel: [w2381 _] -> w2378
                                frame #0 {
                                n275 = call "configuration.vi"("command"="get") -> ("config out"=w2393:T13)  [unwired: 2 in, 1 out]
                                n276 = call "waveformparamsv2.vi"("command"="get") -> ("Params out"=w2387:T16)  [unwired: 4 in, 2 out]
                                n277 = Unbundle By Name(w2393) -> ("Voltage to Xgalvo"=w2394:i32)
                                n278 = call "2pparameters.vi"("command"="get") -> ("params out"=w2390:T12)  [unwired: 1 in]
                                n279 = Unbundle By Name(w2387) -> ("AO parameters"=w2386:T17)
                                n280 = Unbundle By Name(w2390) -> ("aAO"=w2391:u32[])
                                n281 = call "waveformsAObuffer.vi"("command"="get") -> ("AO wf out"=w2383:waveform(dbl)[])  [unwired: 1 in]
                                n282 = Search 1D Array(1D array=w2391, element=w2394) -> (index of element=w2382:i32)  [unwired: 1 in]
                                n283 = Index Array(array=w2383, index=w2382) -> (element=w2381:waveform(dbl))
                                n284 = Index Array(array=w2386, index=w2382) -> (element=w2385:T18)
                                }
                                frame #1 {
                                w2396 = 0.0 ("Step size (V)")
                                n285 = local read "Sampling rate"() -> (w2397:dbl)
                                n286 = call "replace AO XYwfparam.vi"("Baseline (V)"=w2396, "Start amplitude (V)"=w2396, "Cycles"=w2396, "Repeats"=w2396, "index of AO wave"=w2395, "Step size (V)"=w2396, "DC (%)"=w2396, "Sampling frequency (Hz)"=w2397, "Period (ms)"=w2396, "Cycle length (s)"=w2396, "Pulses"=w2396, "padding value"=w2396, "Matlab wave name"=path "xwave") -> ()  [unwired: 3 in]
                                }
                                }
                                }
                                frame True {
                                w2400 = 0.0 ("Repeats")
                                n287 = local read "Sampling rate"() -> (w2409:dbl)
                                n288 = call "2pparameters.vi"("command"="get") -> ("params out"=w2403:T12)  [unwired: 1 in]
                                n289 = call "configuration.vi"("command"="get") -> ("config out"=w2406:T13)  [unwired: 2 in, 1 out]
                                n290 = call "waveformparamsv2.vi"("command"="get") -> ("Params out"=w2415:T16)  [unwired: 4 in, 2 out]
                                n291 = Unbundle By Name(w2406) -> ("Voltage to Xgalvo"=w2407:i32)
                                n292 = Unbundle By Name(w2415) -> ("AO parameters"=w2412:T17)
                                n293 = Unbundle By Name(w2403) -> ("aAO"=w2404:u32[])
                                n294 = Search 1D Array(1D array=w2404, element=w2407) -> (index of element=w2401:i32)  [unwired: 1 in]
                                n295 = Index Array(array=w2412, index=0) -> (element=w2413:T18)
                                n296 = Bundle By Name(cluster=w2413, "AOtab"=-1.0 ("Repeats"), "Repeats"=w2400, "Cycles"=w2400, "Start amplitude (V)"=w2400, "Baseline (V)"=w2400, "Step size (V)"=w2400, "DC (%)"=w2400, "Sampling frequency (Hz)"=w2409, "Period (ms)"=w2400, "Offset (V)"=w2400, "Amplitude (V)"=w2400, "Frequency"=w2400, "Tri Repeats"=w2400, "phase shift (ms)"=w2400, "Pulses"=w2400, "Matlab wave file"=path "xwave", "padding value"=w2400) -> (w2399:T18)
                                n297 = Build Array(w2399) -> (w2410:T17)
                                n298 = call "waveformparamsv2.vi"("command"="add AO", "add AO"=w2410) -> ()  [unwired: 3 in, 3 out]
                                }
                                }
                              }
                              frame #3 {
                                n299 = case shown="False" w2421 {
                                tunnel: [w2424 w2445] -> w2420
                                tunnel: [w2423 w2443] -> w2419
                                tunnel: [w2422 _] -> w2418
                                frame False {
                                n300 = stacked-sequence {
                                seq-local: [w2426 _] -> [_ w2439]
                                tunnel: [w2426 _] -> w2424
                                tunnel: [w2429 _] -> w2423
                                tunnel: [w2425 _] -> w2422
                                frame #0 {
                                n301 = call "configuration.vi"("command"="get") -> ("config out"=w2437:T13)  [unwired: 2 in, 1 out]
                                n302 = call "waveformparamsv2.vi"("command"="get") -> ("Params out"=w2431:T16)  [unwired: 4 in, 2 out]
                                n303 = Unbundle By Name(w2437) -> ("Voltage to Ygalvo"=w2438:i32)
                                n304 = call "2pparameters.vi"("command"="get") -> ("params out"=w2434:T12)  [unwired: 1 in]
                                n305 = Unbundle By Name(w2431) -> ("AO parameters"=w2430:T17)
                                n306 = Unbundle By Name(w2434) -> ("aAO"=w2435:u32[])
                                n307 = call "waveformsAObuffer.vi"("command"="get") -> ("AO wf out"=w2427:waveform(dbl)[])  [unwired: 1 in]
                                n308 = Search 1D Array(1D array=w2435, element=w2438) -> (index of element=w2426:i32)  [unwired: 1 in]
                                n309 = Index Array(array=w2427, index=w2426) -> (element=w2425:waveform(dbl))
                                n310 = Index Array(array=w2430, index=w2426) -> (element=w2429:T18)
                                }
                                frame #1 {
                                w2440 = 0.0 ("Step size (V)")
                                n311 = local read "Sampling rate"() -> (w2441:dbl)
                                n312 = call "replace AO XYwfparam.vi"("Baseline (V)"=w2440, "Start amplitude (V)"=w2440, "Cycles"=w2440, "Repeats"=w2440, "index of AO wave"=w2439, "Step size (V)"=w2440, "DC (%)"=w2440, "Sampling frequency (Hz)"=w2441, "Period (ms)"=w2440, "Cycle length (s)"=w2440, "Pulses"=w2440, "padding value"=w2440, "Matlab wave name"=path "ywave") -> ()  [unwired: 3 in]
                                }
                                }
                                }
                                frame True {
                                w2444 = 0.0 ("Repeats")
                                n313 = local read "Sampling rate"() -> (w2454:dbl)
                                n314 = call "2pparameters.vi"("command"="get") -> ("params out"=w2447:T12)  [unwired: 1 in]
                                n315 = call "configuration.vi"("command"="get") -> ("config out"=w2450:T13)  [unwired: 2 in, 1 out]
                                n316 = call "waveformparamsv2.vi"("command"="get") -> ("Params out"=w2460:T16)  [unwired: 4 in, 2 out]
                                n317 = Unbundle By Name(w2450) -> ("Voltage to Ygalvo"=w2451:i32)
                                n318 = Unbundle By Name(w2460) -> ("AO parameters"=w2457:T17)
                                n319 = Unbundle By Name(w2447) -> ("aAO"=w2448:u32[])
                                n320 = Search 1D Array(1D array=w2448, element=w2451) -> (index of element=w2445:i32)  [unwired: 1 in]
                                n321 = Index Array(array=w2457, index=0) -> (element=w2458:T18)
                                n322 = Bundle By Name(cluster=w2458, "AOtab"=-1.0 ("Repeats"), "Repeats"=w2444, "Cycles"=w2444, "Start amplitude (V)"=w2444, "Baseline (V)"=w2444, "Step size (V)"=w2444, "DC (%)"=w2444, "Sampling frequency (Hz)"=w2454, "Period (ms)"=w2444, "Offset (V)"=w2444, "Amplitude (V)"=w2444, "Frequency"=w2444, "Tri Repeats"=w2444, "phase shift (ms)"=w2444, "Pulses"=w2444, "Matlab wave file"=path "ywave", "padding value"=w2444) -> (w2443:T18)
                                n323 = Build Array(w2443) -> (w2455:T17)
                                n324 = call "waveformparamsv2.vi"("command"="add AO", "add AO"=w2455) -> ()  [unwired: 3 in, 3 out]
                                }
                                }
                              }
                              frame #4 {
                                n325 = call "2pparameters.vi"("command"="get") -> ("params out"=w2467:T12)  [unwired: 1 in]
                                n326 = Unbundle By Name(w2467) -> ("wavdet"=w2466:bool, "sAOxy"=w2463:i32, "refwfsize"=w2462:dbl, "srate Img"=w2465:sgl)
                                n327 = case shown="False" w2466 {
                                tunnel: [w2471 w2481] -> w2469
                                tunnel: w2465 -> [w2472 w2483]
                                tunnel: w2463 -> [_ w2479]
                                tunnel: w2462 -> [_ w2478]
                                frame False {
                                n328 = call "X-array-databuffer.vi"("command"=enum16{"get", "set", "clear", "append"}."get") -> ("array out"=w2475:dbl[])  [unwired: 3 in, 1 out]
                                n329 = Reciprocal(x=w2472) -> (1/x=w2473:sgl)
                                n330 = Bundle By Name("Y"=w2475, "dt"=w2473) -> (w2471:waveform(dbl))  [unwired: 1 in]
                                }
                                frame True {
                                n331 = To Double Precision Float(number=w2479) -> (double precision float=w2480:dbl)
                                n332 = Divide(x=w2478, y=w2480) -> (x/y=w2476:dbl)
                                n333 = Round Toward +Infinity(x=w2476) -> (ceil(x): smallest int >= x=w2477:dbl)
                                n334 = call "X-array-databuffer.vi"("command"=enum16{"get", "set", "clear", "append"}."get") -> ("array out"=w2485:dbl[])  [unwired: 3 in, 1 out]
                                n335 = Reciprocal(x=w2483) -> (1/x=w2484:sgl)
                                n336 = for {
                                N: w2477 -> [_]
                                tunnel: w2485 -> [w2487]
                                tunnel: [w2487] -> w2482 mode=concatenating
                                }
                                n337 = Bundle By Name("Y"=w2482, "dt"=w2484) -> (w2481:waveform(dbl))  [unwired: 1 in]
                                }
                                }
                                n338 = case shown="False" w2470 {
                                tunnel: w2469 -> [w2489 w2495]
                                tunnel: w2464 -> [w2490 _]
                                frame False {
                                n339 = call "waveformsAObuffer.vi"("command"="get") -> ("AO wf out"=w2493:waveform(dbl)[])  [unwired: 1 in]
                                n340 = Replace Array Subset(array=w2493, new element=w2489, index=w2490) -> (w2488:waveform(dbl)[])
                                n341 = call "waveformsAObuffer.vi"("AO wf in"=w2488, "command"="set") -> ()  [unwired: 1 out]
                                }
                                frame True {
                                n342 = call "waveformsAObuffer.vi"("command"="get") -> ("AO wf out"=w2497:waveform(dbl)[])  [unwired: 1 in]
                                n343 = Build Array (concatenate)(w2497, w2495) -> (w2494:waveform(dbl)[])
                                n344 = call "waveformsAObuffer.vi"("AO wf in"=w2494, "command"="set") -> ()  [unwired: 1 out]
                                }
                                }
                              }
                              frame #5 {
                                n345 = call "2pparameters.vi"("command"="get") -> ("params out"=w2509:T12)  [unwired: 1 in]
                                n346 = Unbundle By Name(w2509) -> ("wavdet"=w2508:bool, "sAOxy"=w2506:i32, "refwfsize"=w2507:dbl, "srate Img"=w2502:sgl)
                                n347 = To Double Precision Float(number=w2506) -> (double precision float=w2505:dbl)
                                n348 = Divide(x=w2507, y=w2505) -> (x/y=w2504:dbl)
                                n349 = Round Toward +Infinity(x=w2504) -> (ceil(x): smallest int >= x=w2503:dbl)
                                n350 = case shown="True" w2508 {
                                tunnel: [w2513 w2518] -> w2499
                                tunnel: w2503 -> [_ w2522]
                                tunnel: w2502 -> [w2514 w2520]
                                frame False {
                                n351 = call "Y-array-databuffer.vi"("command"=enum16{"get", "set", "clear", "append"}."get") -> ("array out"=w2511:dbl[])  [unwired: 3 in, 1 out]
                                n352 = Reciprocal(x=w2514) -> (1/x=w2515:sgl)
                                n353 = Bundle By Name("Y"=w2511, "dt"=w2515) -> (w2513:waveform(dbl))  [unwired: 1 in]
                                }
                                frame True {
                                n354 = call "Y-array-databuffer.vi"("command"=enum16{"get", "set", "clear", "append"}."get") -> ("array out"=w2516:dbl[])  [unwired: 3 in, 1 out]
                                n355 = Reciprocal(x=w2520) -> (1/x=w2521:sgl)
                                n356 = for {
                                N: w2522 -> [_]
                                tunnel: w2516 -> [w2523]
                                tunnel: [w2523] -> w2519 mode=concatenating
                                }
                                n357 = Bundle By Name("Y"=w2519, "dt"=w2521) -> (w2518:waveform(dbl))  [unwired: 1 in]
                                }
                                }
                                n358 = case shown="False" w2501 {
                                tunnel: w2499 -> [w2526 w2531]
                                tunnel: w2500 -> [w2527 _]
                                frame False {
                                n359 = call "waveformsAObuffer.vi"("command"="get") -> ("AO wf out"=w2529:waveform(dbl)[])  [unwired: 1 in]
                                n360 = Replace Array Subset(array=w2529, new element=w2526, index=w2527) -> (w2524:waveform(dbl)[])
                                n361 = call "waveformsAObuffer.vi"("AO wf in"=w2524, "command"="set") -> ()  [unwired: 1 out]
                                }
                                frame True {
                                n362 = call "waveformsAObuffer.vi"("command"="get") -> ("AO wf out"=w2533:waveform(dbl)[])  [unwired: 1 in]
                                n363 = Build Array (concatenate)(w2533, w2531) -> (w2530:waveform(dbl)[])
                                n364 = call "waveformsAObuffer.vi"("AO wf in"=w2530, "command"="set") -> ()  [unwired: 1 out]
                                }
                                }
                              }
                              frame #6 {
                                n365 = Build Array(w2538, w2537) -> (w2541:bool[])
                                n366 = Boolean Array To Number(Boolean array=w2541) -> (number=w2540:u32)
                                n367 = case shown="0" w2540 {
                                tunnel: w2539 -> [_ _ _ _]
                                tunnel: w2536 -> [_ w2564 _ w2577]
                                tunnel: [_ w2563 _ w2574] -> w2535
                                frame 1 {
                                w2551 = 0.0 ("DOtab")
                                n368 = call "2pparameters.vi"("command"="get") -> ("params out"=w2548:T12)  [unwired: 1 in]
                                n369 = call "waveformparamsv2.vi"("command"="get") -> ("Params out"=w2559:T16)  [unwired: 4 in, 2 out]
                                n370 = Unbundle By Name(w2559) -> ("DO parameters"=w2557:T19)
                                n371 = Unbundle By Name(w2548) -> ("srate"=w2544:sgl, "sAOxy"=w2547:i32)
                                n372 = To Double Precision Float(number=w2544) -> (double precision float=w2542:dbl)
                                n373 = To Double Precision Float(number=w2544) -> (double precision float=w2543:dbl)
                                n374 = To Double Precision Float(number=w2547) -> (double precision float=w2546:dbl)
                                n375 = Divide(x=w2543, y=w2546) -> (x/y=w2545:dbl)
                                n376 = Index Array(array=w2557, index=0) -> (element=w2556:T20)
                                n377 = Bundle By Name(cluster=w2556, "Digital DC (%)"=100.0, "Digital phase"=w2551, "Digital Freq (Hz)"=w2545, "Sampling frequency (Hz)"=w2542, "Digital time offset (s)"=w2551, "padding value"=0.0, "matlab wave file"=path "2Pshutter", "DOtab"=0.0) -> (w2554:T20)
                                n378 = Build Array(w2554) -> (w2553:T19)
                                n379 = call "waveformparamsv2.vi"("command"="add DO", "add DO"=w2553) -> ()  [unwired: 3 in, 3 out]
                                }
                                frame 2 {
                                n380 = call "waveformparamsv2.vi"("command"="get") -> ("Params out"=w2566:T16)  [unwired: 4 in, 2 out]
                                n381 = in-place {
                                in-place-border: w2564 -> [w2570]
                                in-place-border: [w2569] -> w2563
                                n382 = in-place-cluster #7(w2566) -> ("DO parameters"=w2572:T19)
                                n383 = Delete From Array(array=w2572, length=1, index=w2570) -> (deleted portion=w2569:T19, array with subset deleted=w2571:T19)
                                n384 = in-place-cluster #7("DO parameters"=w2571) -> (w2565:T16)
                                }
                                n385 = call "waveformparamsv2.vi"("command"="set", "Params in"=w2565) -> ()  [unwired: 3 in, 3 out]
                                }
                                frame 3, Default {
                                }
                                frame 0 {
                                n386 = call "2pparameters.vi"("command"="get") -> ("params out"=w2579:T12)  [unwired: 1 in]
                                n387 = Unbundle By Name(w2579) -> ("wavdet"=w2576:bool, "autoshutter"=w2578:bool)
                                n388 = case shown="True" w2578 {
                                tunnel: w2577 -> [_ w2583]
                                tunnel: w2576 -> [_ w2582]
                                tunnel: [_ w2581] -> w2575
                                frame False {
                                }
                                frame True {
                                n389 = case shown="False" w2582 {
                                tunnel: w2583 -> [w2585 _]
                                tunnel: [w2584 _] -> w2581
                                frame False {
                                n390 = stacked-sequence {
                                tunnel: w2585 -> [w2587 w2601]
                                tunnel: [w2586 _] -> w2584
                                frame #0 {
                                n391 = call "waveformparamsv2.vi"("command"="get") -> ("Params out"=w2589:T16)  [unwired: 4 in, 2 out]
                                n392 = Unbundle By Name(w2589) -> ("DO parameters"=w2588:T19)
                                n393 = Index Array(array=w2588, index=w2587) -> (element=w2586:T20)
                                }
                                frame #1 {
                                w2600 = 0.0 ("padding value")
                                n394 = call "2pparameters.vi"("command"="get") -> ("params out"=w2598:T12)  [unwired: 1 in]
                                n395 = Unbundle By Name(w2598) -> ("srate"=w2595:sgl, "sAOxy"=w2597:i32)
                                n396 = To Double Precision Float(number=w2595) -> (double precision float=w2593:dbl)
                                n397 = To Double Precision Float(number=w2595) -> (double precision float=w2594:dbl)
                                n398 = To Double Precision Float(number=w2597) -> (double precision float=w2596:dbl)
                                n399 = Divide(x=w2594, y=w2596) -> (x/y=w2592:dbl)
                                n400 = call "replace DO wf param.vi"("Digital Freq (Hz)"=w2592, "Digital DC (%)"=100.0, "Digital phase"=w2600, "Sampling frequency (Hz)"=w2593, "Digital time offset (s)"=w2600, "index of DO wave"=w2601, "padding value"=w2600, "matlab wave file"=path "2Pshutter" ("matlab wave number")) -> ()  [unwired: 3 in]
                                }
                                }
                                }
                                frame True {
                                }
                                }
                                }
                                }
                                n401 = Build Array(w2575) -> (w2574:T19)
                                }
                                }
                              }
                              frame #7 {
                                n402 = Build Array(w2606, w2605) -> (w2608:bool[])
